vi "InitCSMs.vi"(8 "error in":errorcluster) -> (0 "error out":errorcluster, 2 "CSMs":string[](array[string]))   [LabVIEW 2017]
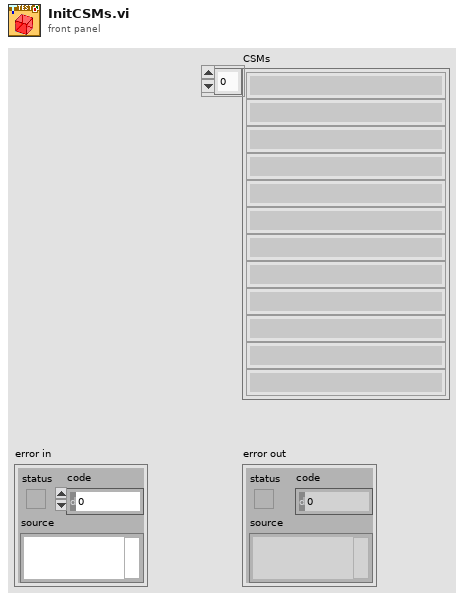
[diagram p1: front panel]
types:
  T1 = cluster{"prototype":string, "name":string, "num":i32, "index":i32}[]
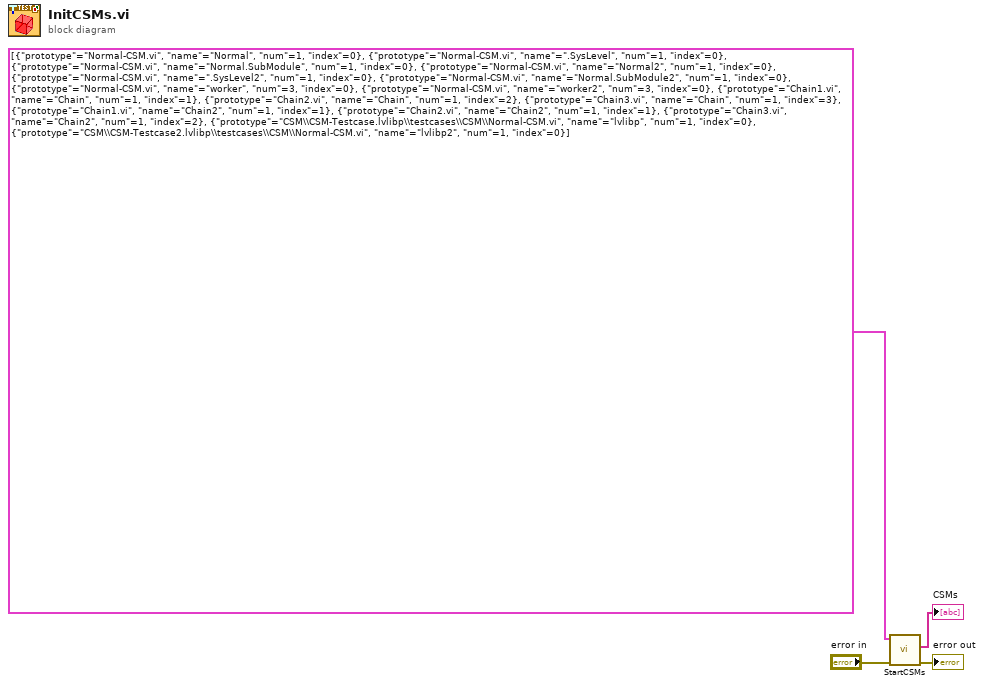
[diagram p0: block diagram]
diagram:
  n1 = call "StartCSMs.vi"("error in"="error in", "Array"=T1 [{"prototype"="Normal-CSM.vi", "name"="Normal", "num"=1, "index"=0}, {"prototype"="Normal-CSM.vi", "name"=".SysLevel", "num"=1, "index"=0}, {"prototype"="Normal-CSM.vi", "name"="Normal.SubModule", "num"=1, "index"=0}, {"prototype"="Normal-CSM.vi", "name"="Normal2", "num"=1, "index"=0}, {"prototype"="Normal-CSM.vi", "name"=".SysLevel2", "num"=1, "index"=0}, {"prototype"="Normal-CSM.vi", "name"="Normal.SubModule2", "num"=1, "index"=0}, {"prototype"="Normal-CSM.vi", "name"="worker", "num"=3, "index"=0}, {"prototype"="Normal-CSM.vi", "name"="worker2", "num"=3, "index"=0}, {"prototype"="Chain1.vi", "name"="Chain", "num"=1, "index"=1}, {"prototype"="Chain2.vi", "name"="Chain", "num"=1, "index"=2}, {"prototype"="Chain3.vi", "name"="Chain", "num"=1, "index"=3}, {"prototype"="Chain1.vi", "name"="Chain2", "num"=1, "index"=1}, {"prototype"="Chain2.vi", "name"="Chain2", "num"=1, "index"=1}, {"prototype"="Chain3.vi", "name"="Chain2", "num"=1, "index"=2}, {"prototype"="CSM\\CSM-Testcase.lvlibp\\testcases\\CSM\\Normal-CSM.vi", "name"="lvlibp", "num"=1, "index"=0}, {"prototype"="CSM\\CSM-Testcase2.lvlibp\\testcases\\CSM\\Normal-CSM.vi", "name"="lvlibp2", "num"=1, "index"=0}]) -> ("error out"=→"error out":errorcluster, "CSMs"=→"CSMs":string[])  [unwired: 8 in]
